vi "Create Gradient Array.vi"(8 "Values to Include":enum16{"Start", "End", "Start and End", "None"}(ring)=enum."Start and End", 9 "Array Length":dbl, 10 "End Value":dbl, 11 "Start Value":dbl) -> (3 "Output Array":dbl[](array[numeric]))   [LabVIEW 2020, in "Graphics.lvclass"]
doc: "This VI will create an array of gradient values starting at the specified value, ending at the specified value, and having the number of steps specified.\n\nhttps://decibel.ni.com/content/docs/DOC-9294\n\n-----\nBrian Hoover (hooovahh)"
uses:
  <resource>/Framework/Providers/Open_GDS/UML/Graphics_class/Graphics.lvclass
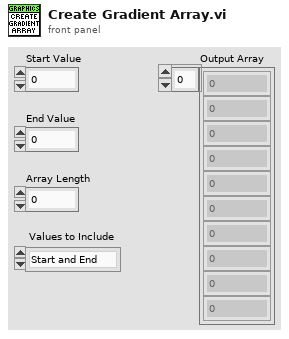
[diagram p1: front panel]
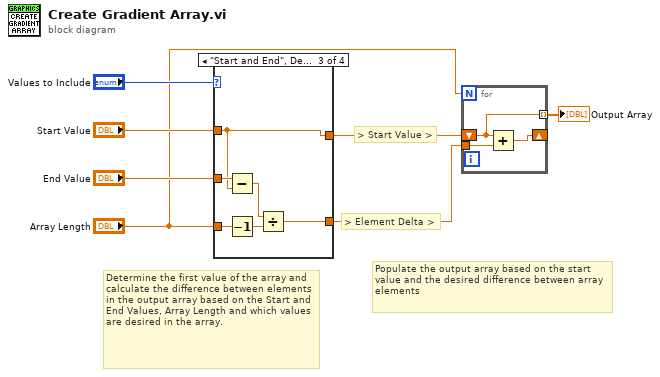
[diagram p0: block diagram]
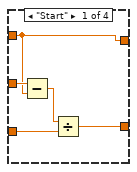
[diagram p2: hidden frame]
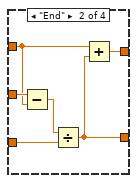
[diagram p3: hidden frame]
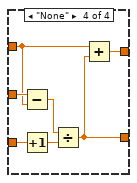
[diagram p4: hidden frame]
diagram:
  # "Populate the output array based on the start value and the desired difference between array elements"
  # "> Element Delta >"
  # "> Start Value >"
  # "Determine the first value of the array and calculate the difference between elements in the output array based on the Start and End Values, Array Length and which values are desired in the array."
  n1 = case shown="\"Start and End\", Default" "Values to Include" {
    tunnel: "End Value" -> [w10 w17 w21 w29]
    tunnel: [w11 w15 w22 w26] -> w6
    tunnel: "Array Length" -> [w9 w16 w20 w28]
    tunnel: "Start Value" -> [w8 w13 w19 w25]
    tunnel: [w8 w14 w19 w27] -> w3
    frame "Start" {
      n2 = Subtract(x=w10, y=w8) -> (x-y=w12:dbl)
      n3 = Divide(x=w12, y=w9) -> (x/y=w11:dbl)
    }
    frame "End" {
      n4 = Subtract(x=w17, y=w13) -> (x-y=w18:dbl)
      n5 = Divide(x=w18, y=w16) -> (x/y=w15:dbl)
      n6 = Add(x=w13, y=w15) -> (x+y=w14:dbl)
    }
    frame "Start and End", Default {
      n7 = Subtract(x=w21, y=w19) -> (x-y=w24:dbl)
      n8 = Decrement(x=w20) -> (x-1=w23:dbl)
      n9 = Divide(x=w24, y=w23) -> (x/y=w22:dbl)
    }
    frame "None" {
      n10 = Subtract(x=w29, y=w25) -> (x-y=w30:dbl)
      n11 = Increment(x=w28) -> (x+1=w31:dbl)
      n12 = Divide(x=w30, y=w31) -> (x/y=w26:dbl)
      n13 = Add(x=w25, y=w26) -> (x+y=w27:dbl)
    }
  }
  n14 = for {
    N: "Array Length" -> [_]
    tunnel: w6 -> [w34]
    shift-right: [w33] -> _
    shift-left: w3 -> [w32]
    tunnel: [w32] -> w1 mode=indexing
    n15 = Add(x=w32, y=w34) -> (x+y=w33:dbl)
  }
  "Output Array" <- w1
